vi "writeI16.vi"(8 "error in (no error)":errorcluster, 10 "Input":i16, 11 "ModbusBuffer in":refnum<class "ModbusBufferBuilder.lvclass">) -> (0 "error out":errorcluster, 3 "ModbusBuffer out":refnum<class "ModbusBufferBuilder.lvclass">)   [LabVIEW 2016, in "ModbusBufferBuilder.lvclass"]
uses:
  ModbusBufferBuilder.lvclass
  ModbusBufferBuilder.lvclass/ModbusBufferBuilder.ctl
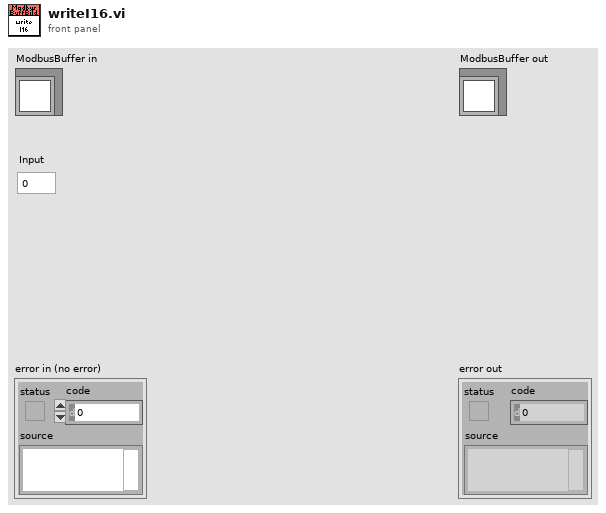
[diagram p1: front panel]
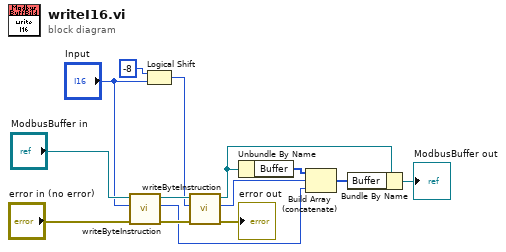
[diagram p0: block diagram]
diagram:
  n1 = call "writeByteInstruction.vi"("error in (no error)"="error in (no error)", "Input"="Input", "ModbusBuffer in"="ModbusBuffer in") -> ("error out"=w8:errorcluster, "Output"=w2:u16, "ModbusBuffer out"=w12:refnum<class "ModbusBufferBuilder.lvclass">)  [unwired: 6 in]
  n2 = Logical Shift(y=i16 -8, x="Input") -> (x << y=w10:i16)
  n3 = call "writeByteInstruction.vi"("error in (no error)"=w8, "Input"=w10, "ModbusBuffer in"=w12) -> ("error out"=→"error out":errorcluster, "Output"=w3:u16, "ModbusBuffer out"=w7:refnum<class "ModbusBufferBuilder.lvclass">)  [unwired: 6 in]
  n4 = Unbundle By Name(w7) -> ("Buffer"=w4:u16[])
  n5 = Build Array (concatenate)(w4, w3, w2) -> (w1:u16[])
  n6 = Bundle By Name(cluster=w7, "Buffer"=w1) -> (→"ModbusBuffer out":refnum<class "ModbusBufferBuilder.lvclass">)
